vi "sub build basic data.vi"(8 "error in":errorcluster, 11 "frame basic data":T1) -> (0 "error out":errorcluster, 3 "basic string":string)   [LabVIEW 2018, in "Data Parser.lvclass"]
uses:
  Data Parser.lvclass
  frame basic data.ctl
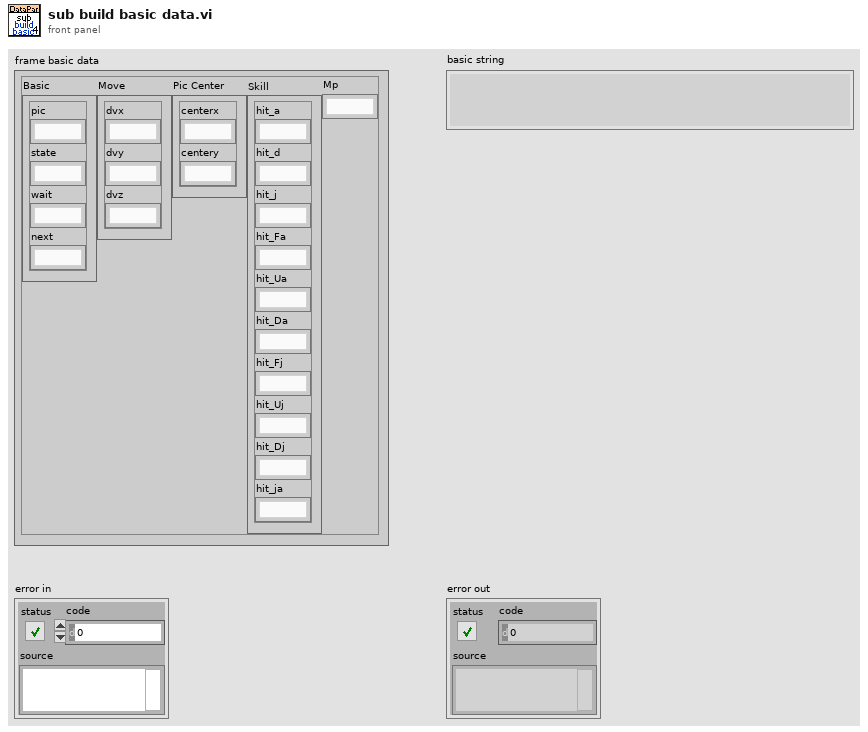
[diagram p1: front panel]
types:
  T1 = typedef "Data Parser.lvclass/frame basic data.ctl" = cluster{"Basic":cluster{"pic":string, "state":string, "wait":string, "next":string}, "Move":cluster{"dvx":string, "dvy":string, "dvz":string}, "Pic Center":cluster{"centerx":string, "centery":string}, "Skill":cluster{"hit_a":string, "hit_d":string, "hit_j":string, "hit_Fa":string, "hit_Ua":string, "hit_Da":string, "hit_Fj":string, "hit_Uj":string, "hit_Dj":string, "hit_ja":string}, "Mp":string}
  T2 = cluster{"pic":string, "state":string, "wait":string, "next":string}
  T3 = cluster{"dvx":string, "dvy":string, "dvz":string}
  T4 = cluster{"hit_a":string, "hit_d":string, "hit_j":string, "hit_Fa":string, "hit_Ua":string, "hit_Da":string, "hit_Fj":string, "hit_Uj":string, "hit_Dj":string, "hit_ja":string}
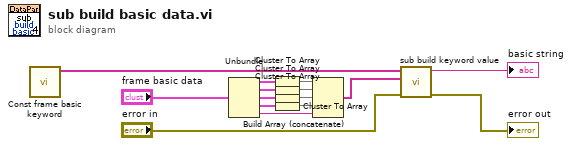
[diagram p0: block diagram]
diagram:
  n1 = call "Const frame basic keyword.vi"() -> ("Const frame basic keyword"=w5:string[])  [unwired: 11 in]
  n2 = Unbundle("frame basic data") -> ("Basic"=w14:T2, "Move"=w13:T3, "Pic Center"=w12:cluster{"centerx":string, "centery":string}, "Skill"=w4:T4, "Mp"=w2:string)
  n3 = Cluster To Array(cluster=w14) -> (array=w11:string[])
  n4 = Cluster To Array(cluster=w13) -> (array=w10:string[])
  n5 = Cluster To Array(cluster=w12) -> (array=w9:string[])
  n6 = Cluster To Array(cluster=w4) -> (array=w3:string[])
  n7 = Build Array (concatenate)(w11, w10, w9, w3, w2) -> (w1:string[])
  n8 = call "sub build keyword value.vi"("error in"="error in", "value"=w1, "keyword"=w5) -> ("error out"=→"error out":errorcluster, "keyword value string"=→"basic string":string)  [unwired: 7 in]
